vi "Formate Assertions for Description.vi"(10 "Item":string, 11 "Result Model in":refnum<class "Result Model.lvclass">) -> (2 "Assertions Description":string)   [LabVIEW 2020, in "Result Model.lvclass"]
uses:
  Result Model.lvclass
  Result Model.lvclass/Result Model.ctl
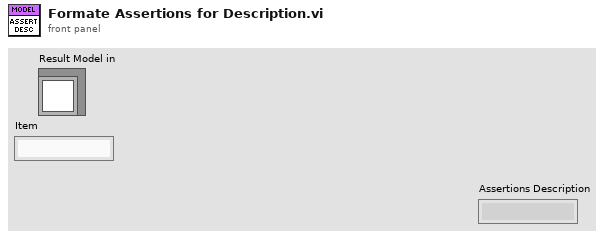
[diagram p1: front panel]
types:
  T1 = typedef "Result Model.lvclass/Model State.ctl" = cluster{"Run Queue":set{string}, "Test Statuses":map{string, T2}, "Execution Time":map{string, dbl}, "Assertions":map{string, cluster{"Result Type":T3, "Status":T2, "Message":string, "Description":string}[]}}
  T2 = typedef "Result.lvlib/Status.ctl" = enum16{"", "Passed", "Failed", "Error", "Skipped", "Setup Error", "Broken", "Teardown Error"}
  T3 = typedef "Result.lvlib/Type.ctl" = enum16{"Method", "Case", "Suite", "Pass", "Fail", "Skip", "Pass if", "Fail if", "Pass if Error", "Fail if Error", "Pass if Equal", "Fail if Equal"}
  T4 = map{string, cluster{"Result Type":T3, "Status":T2, "Message":string, "Description":string}[]}
  T5 = cluster{"Result Type":T3, "Status":T2, "Message":string, "Description":string}[]
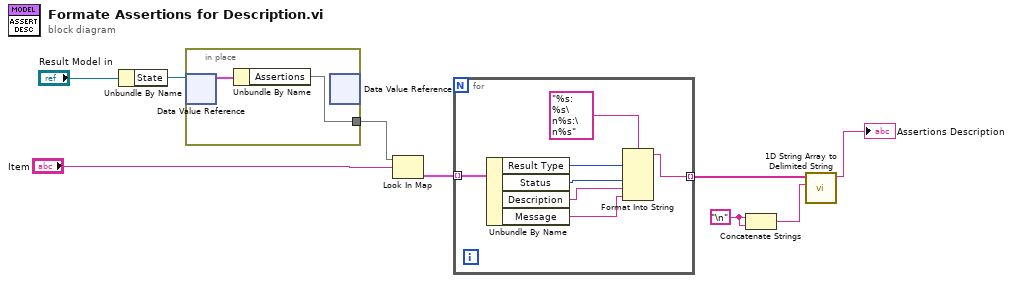
[diagram p0: block diagram]
diagram:
  w4 = "\n"
  n1 = Unbundle By Name("Result Model in") -> ("State"=w2:refnum<data-value>)
  n2 = in-place {
    in-place-border: [w10] -> w1
    n3 = in-place-dvr #1(w2) -> (w11:T1)  [unwired: 1 out]
    n4 = Unbundle By Name(w11) -> ("Assertions"=w10:T4)
    n5 = in-place-dvr #1() -> ()  [unwired: 1 in, 2 out]
  }
  n6 = Look In Map(map=w1, key="Item") -> (value=w6:T5)  [unwired: 1 in, 1 out]
  n7 = for {
    tunnel: [w17] -> w9 mode=indexing
    tunnel: w6 -> [w14] mode=indexing
    n8 = Unbundle By Name(w14) -> ("Result Type"=w16:T3, "Status"=w15:T2, "Description"=w13:string, "Message"=w12:string)
    n9 = Format Into String(format string="%s: %s\n%s:\n%s", w16, w15, w13, w12) -> (resulting string=w17:string)  [unwired: 2 in, 1 out]
  }
  n10 = Concatenate Strings(w4, w4) -> (w5:string)
  n11 = call <vilib>:"1D String Array to Delimited String.vi"("delimiter"=w5, "string array"=w9) -> ("delimited string"=→"Assertions Description":string)  [unwired: 9 in]
